vi "meas_BOC_RMS.vi"(8 "error in (no error)":errorcluster, 11 "output cluster in":T1) -> (0 "error out":errorcluster, 1 "boc_data":sgl[](array[numeric]), 2 "meas":dbl[](array[numeric]), 3 "output cluster out":T1)   [LabVIEW 2017]
uses:
  controls/app_data.ctl
  controls/instruments.ctl
  Unicorn Labview Library/Control/unicorn_Param.ctl
  Unicorn Labview Library/Control/unicorn_conn.ctl
  Unicorn Labview Library/Control/unicorn_JSON.ctl
  Unicorn Labview Library/Control/unicorn_ParamInt.ctl
  Unicorn Labview Library/Control/unicorn_Telemetry.ctl
  Unicorn Labview Library/Control/unicorn_Table.ctl
  Unicorn Labview Library/Control/unicorn_ParamFloat.ctl
  <instrlib>/PICOTEST M352XA/Public/Controls/Function.ctl
  Unicorn Labview Library/Unicorn Library.lvlib
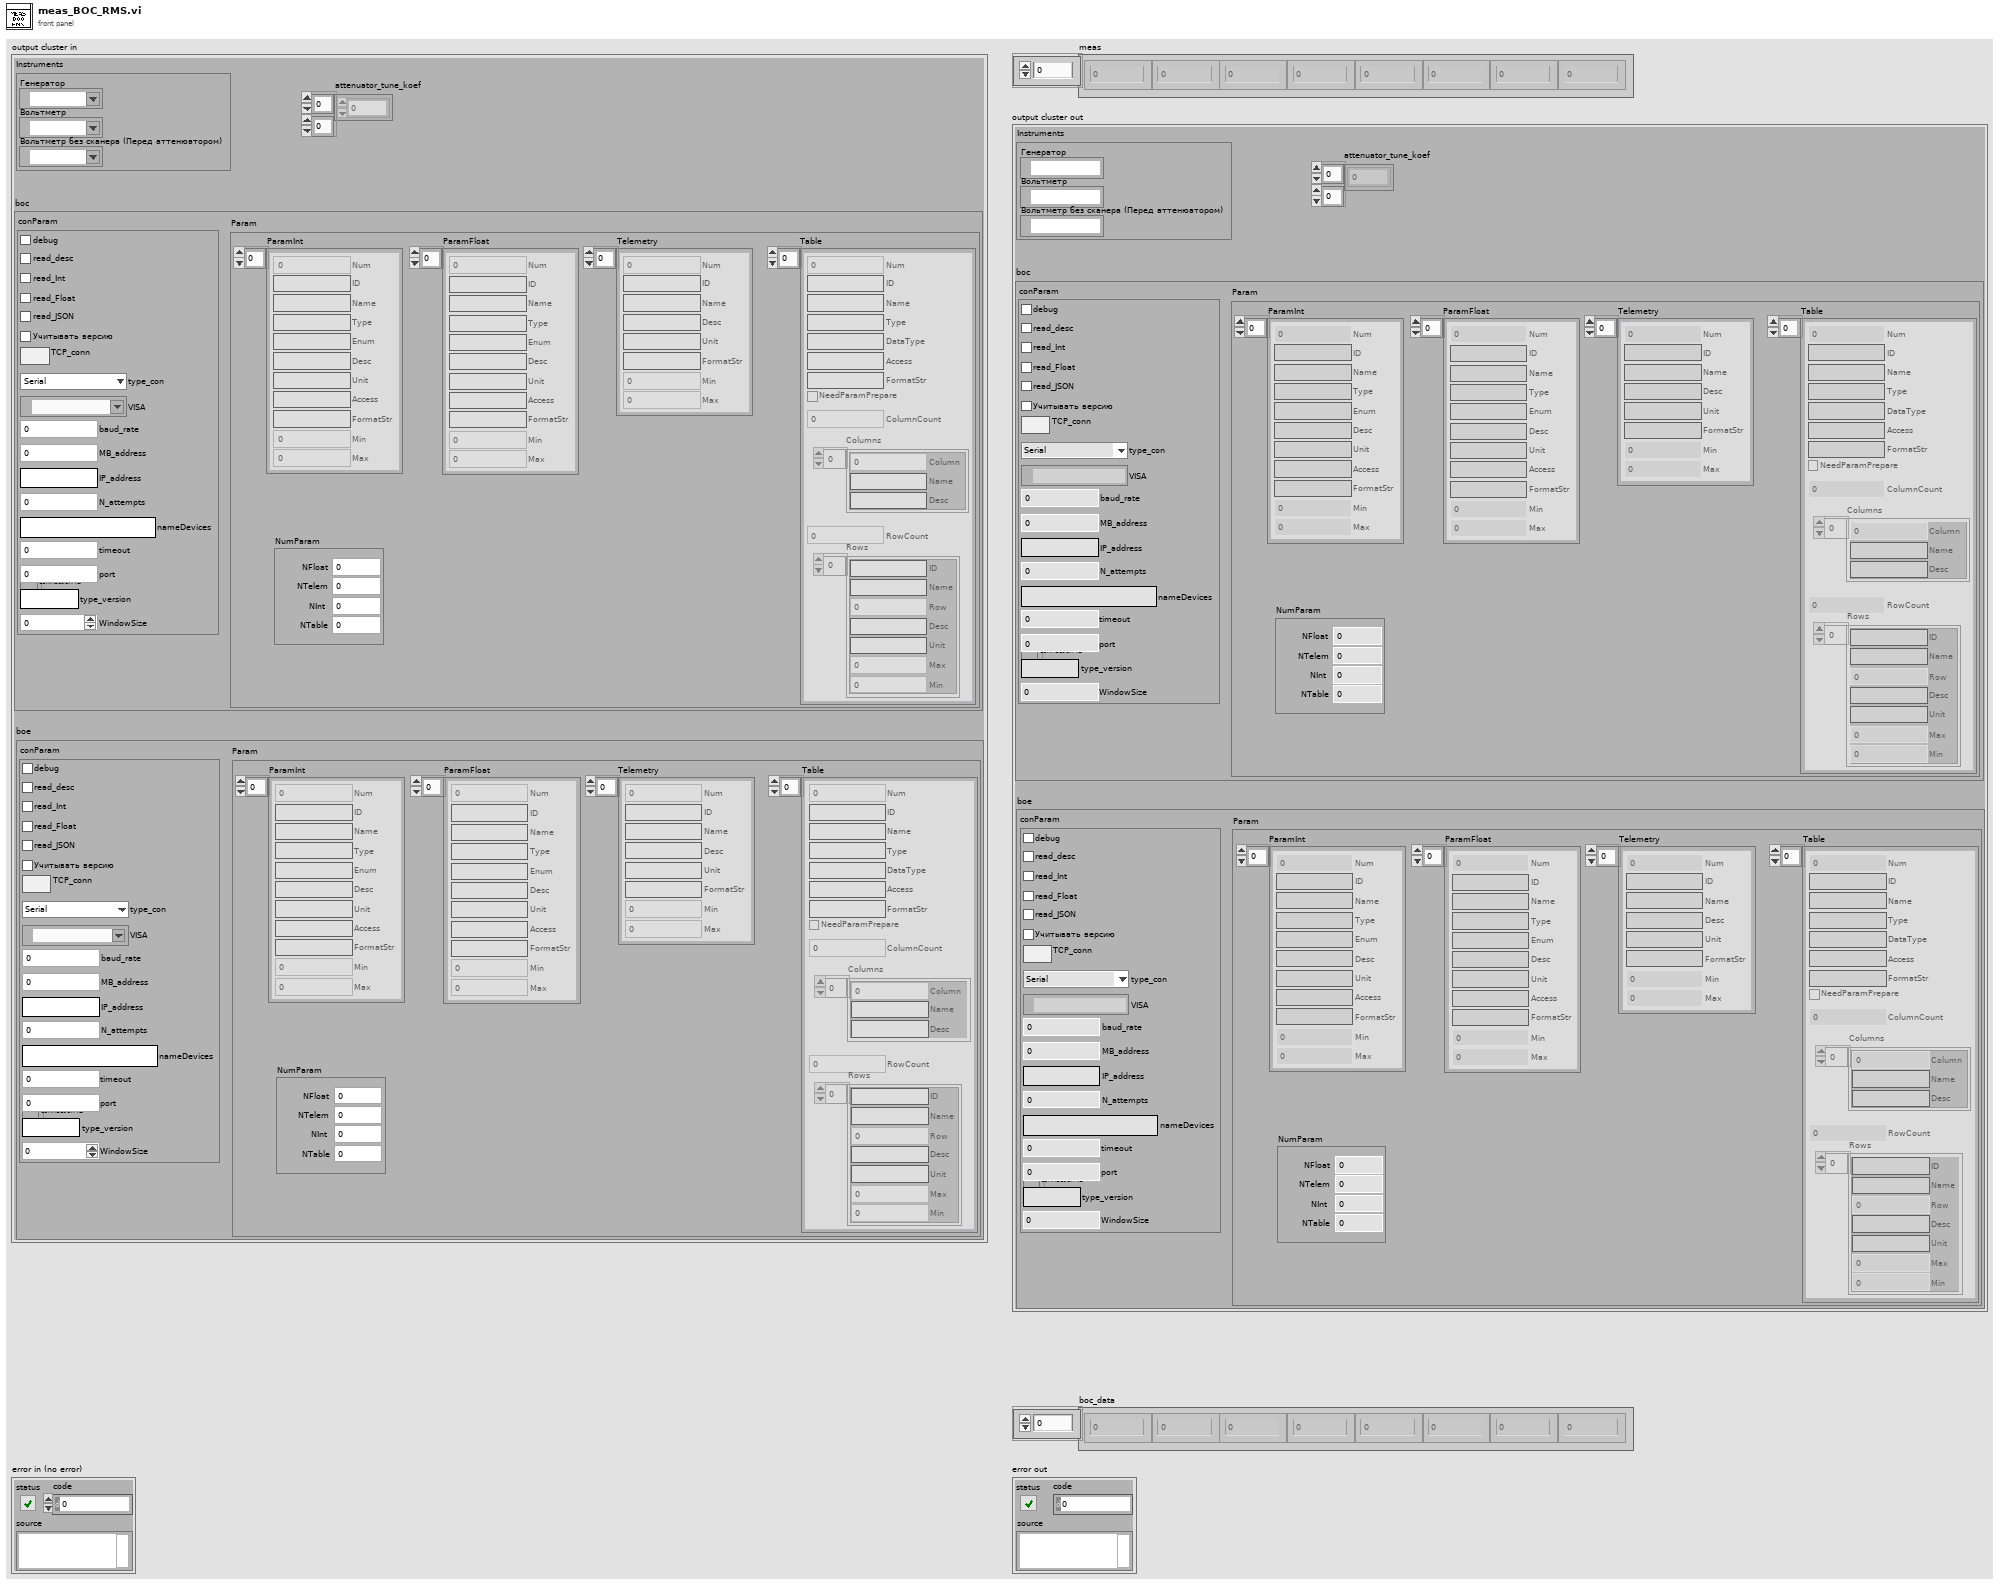
[diagram p1: front panel]
types:
  T1 = typedef "app_data.ctl" = cluster{"Instruments":T2, "boc":T3, "boe":T3, "attenuator_tune_koef":dbl[][]}
  T2 = typedef "instruments.ctl" = cluster{"generator":refnum<visa-resource-name>, "voltment_with_scaner":refnum<visa-resource-name>, "voltment_without_scaner":refnum<visa-resource-name>}
  T3 = typedef "Unicorn Library.lvlib/unicorn_Param.ctl" = cluster{"conParam":T4, "Param":T5}
  T4 = typedef "Unicorn Library.lvlib/unicorn_conn.ctl" = cluster{"ReadIntParam":bool, "ReadDescrParam":bool, "ReadFloatParam":bool, "debug":bool, "ReadJSON":bool, "IP_address":string, "N_attempts":i32, "type_con":enum16{"Serial", "TCP"}, "MB_address":i32, "VISA":refnum<visa-resource-name>, "connection ID":refnum<k5>, "nameDevices":string, "timeout":i32, "port":u16, "type_version":string, "baud_rate":u32, "VersionControl":bool, "TCP_conn":bool, "WindowSize":i32}
  T5 = typedef "Unicorn Library.lvlib/unicorn_JSON.ctl" = cluster{"NumParam":cluster{"NTelem":i32, "NInt":i32, "NFloat":i32, "NTable":i32}, "ParamInt":T6, "Telemetry":T7, "Table":T8, "ParamFloat":T9}
  T6 = typedef "Unicorn Library.lvlib/unicorn_ParamInt.ctl" = cluster{"ID":string, "Num":i32, "Name":string, "Type":string, "Enum":string, "Desc":string, "Unit":string, "Access":string, "FormatStr":string, "Min":i32, "Max":i32}[]
  T7 = typedef "Unicorn Library.lvlib/unicorn_Telemetry.ctl" = cluster{"ID":string, "Num":i32, "Name":string, "Desc":string, "Unit":string, "FormatStr":string, "Min":i32, "Max":i32}[]
  T8 = typedef "Unicorn Library.lvlib/unicorn_Table.ctl" = cluster{"Num":i32, "Access":string, "ColumnCount":i32, "NeedParamPrepare":bool, "Columns":cluster{"Column":i32, "Desc":string, "Name":string}[], "DataType":string, "FormatStr":string, "ID":string, "Name":string, "RowCount":i32, "Rows":cluster{"Desc":string, "ID":string, "Max":i32, "Min":i32, "Name":string, "Row":i32, "Unit":string}[], "Type":string}[]
  T9 = typedef "Unicorn Library.lvlib/unicorn_ParamFloat.ctl" = cluster{"ID":string, "Num":i32, "Name":string, "Type":string, "Enum":string, "Desc":string, "Unit":string, "Access":string, "FormatStr":string, "Min":i32, "Max":i32}[]
  T10 = typedef "Function.ctl" = enum16{"VOLTage:DC", "VOLTage:DC:RATio", "VOLTage:AC", "CURRent:DC", "CURRent:AC", "RESistance", "FRESistance", "FREQuency", "PERiod", "FREQuency:CURRent", "PERiod:CURRent", "CAPacitance", "CONTinuity", "DIODe", "TCOuple", "TEMPerature"}
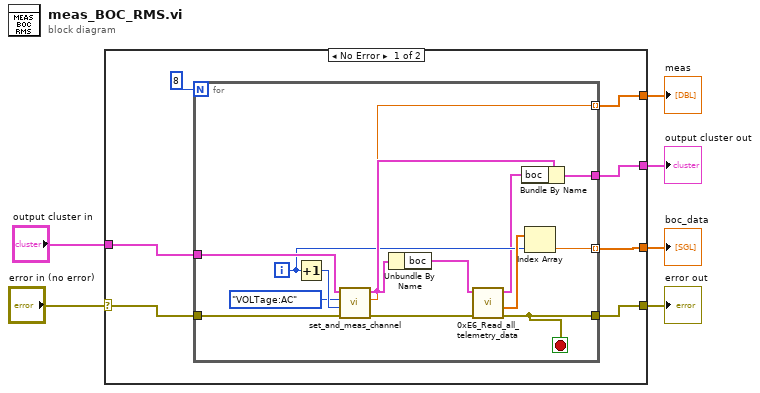
[diagram p0: block diagram]
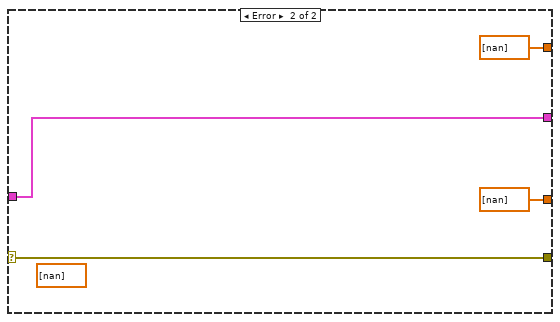
[diagram p2: hidden frame]
diagram:
  n1 = case shown="No Error" "error in (no error)" {
    selector: "error in (no error)" -> [w7 w30]
    tunnel: [w13 w30] -> w6
    tunnel: [w12 dbl[] [nan]] -> w5
    tunnel: [w11 w31] -> w4
    tunnel: [w10 sgl[] [nan]] -> w3
    tunnel: "output cluster in" -> [w9 w31]
    frame No Error {
      n2 = for {
        N: 8 -> [_]
        tunnel: w9 -> [w24]
        tunnel: w7 -> [w26]
        tunnel: [w20] -> w11
        tunnel: [w19] -> w10 mode=indexing
        tunnel: [w16] -> w12 mode=indexing
        tunnel: [w14] -> w13
        i -> [w18]
        stop <- w14 stop-if-true
        n3 = Increment(x=w18) -> (x+1=w25:i32)
        n4 = call "set_and_meas_channel.vi"("error in (no error)"=w26, "channel"=w25, "Function"=Function."VOLTage:AC", "output cluster"=w24) -> ("error out"=w15:errorcluster, "Measurement"=w16:dbl, "output cluster 2"=w21:T1)  [unwired: 5 in]
        n5 = Unbundle By Name(w21) -> ("boc"=w22:T3)
        n6 = call "0xE6_Read_all_telemetry_data.vi"("error in"=w15, "paramUnicorn"=w22) -> ("error out"=w14:errorcluster, "Telemetry"=w27:sgl[], "paramUnicorn 2"=w17:T3)  [unwired: 5 in, 1 out]
        n7 = Bundle By Name(cluster=w21, "boc"=w17) -> (w20:T1)
        n8 = Index Array(array=w27, index=w18) -> (element=w19:sgl)
      }
    }
    frame Error {
      (unwired) dbl[] [nan]
    }
  }
  "boc_data" <- w3
  "meas" <- w5
  "error out" <- w6
  "output cluster out" <- w4
